vi "Main.vi"() -> ()   [LabVIEW 2012]
doc: "DESCRIPTION:\nThe One-Axis Move (Accel - Max Velocity - Decel) VI completes a move to user-specified position on a single axis while using user-specified acceleration, maximum velocity, and deceleration values. It also provides a monitor to track the progress of the move.\n\n*Note: This VI can be used as a subVI in a higher level program.\n\nINSTRUCTIONS:\n(1) Be sure your board is initialized before running this VI. Refer to the Initialization topic in the FlexMotion VI Online Help, which can be launched by choosing FlexMotion VI Online Help in the Help menu.\n\n(2) Select the Board ID that corresponds to your FlexMotion controller in the Board Configuration Utility. \n\n(3) Select the axis number to be used.\n\n(4) Set the Target Position (in encoder counts) to which you want the axis to move.\n\n(5) Set the values you wish to use for maximum velocity (RPM), acceleration (RPS/S), and deceleration (RPS/S).\n\n(6) Run the VI.\n\nKEY PARAMETERS:\n(1) Target Position: The position to which you want to move. This value needs to be changed every time you run the VI. If you run the VI twice in a row with the same target position, the motor will not move the second time since it will already be at its target position.\n\n(2) Velocity: The maximum velocity for the specified axis during the move.\n\n(3) Acceleration: The acceleration for the axis during the move.\n\n(4) Deceleration: The deceleration for the axis during the move. (This may be different than the acceleration.)\n\nI/O CONNECTIONS OVERVIEW:\nThis example requires a system configuration with one axis."
uses:
  MicroDrive.dll
panel:
  in  "Threshold(um)":dbl=0.5 format="%.3f"
  in  "Iterations":i32=1
  out "M6 Forward Limit":bool
  out "M6 Reverse Limit":bool
  out "M5 Forward Limit":bool
  out "M5 Reverse Limit":bool
  out "M4 Forward Limit":bool
  out "M4 Reverse Limit":bool
  in  "Reset M4":bool
  in  "Flip M4 Encoder":bool
  out "M4 Encoder (um)":dbl format="%.3f"
  in  "Flip M3 Encoder":bool
  in  "Flip M2 Encoder":bool
  in  "Flip M1 Encoder":bool
  out "M3 Encoder (um)":dbl format="%.3f"
  in  "Reset M3":bool
  out "M3 Forward Limit":bool
  out "M3 Reverse Limit":bool
  in  "Axis":enum16{"M1", "M2", "M3", "M4", "M5", "M6"}(ring)
  in  "Velocity (mm/s)":dbl=1.0 format="%.3f"
  in  "Move size (um)":dbl=50.0 format="%.3f"
  out "M2 Forward Limit":bool
  out "M2 Reverse Limit":bool
  out "M1 Forward Limit":bool
  out "M1 Reverse Limit":bool
  in  "stop":bool
  out "M2 Encoder (um)":dbl format="%.3f"
  in  "Reset  All":bool
  in  "Reset M2":bool
  out "M1 Encoder (um)":dbl format="%.3f"
  in  "Reset M1":bool
  in  "Move":bool
  in  "Stop":bool
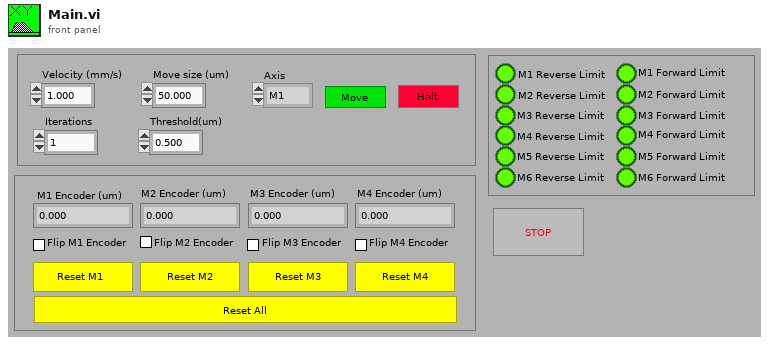
[diagram p1: front panel]
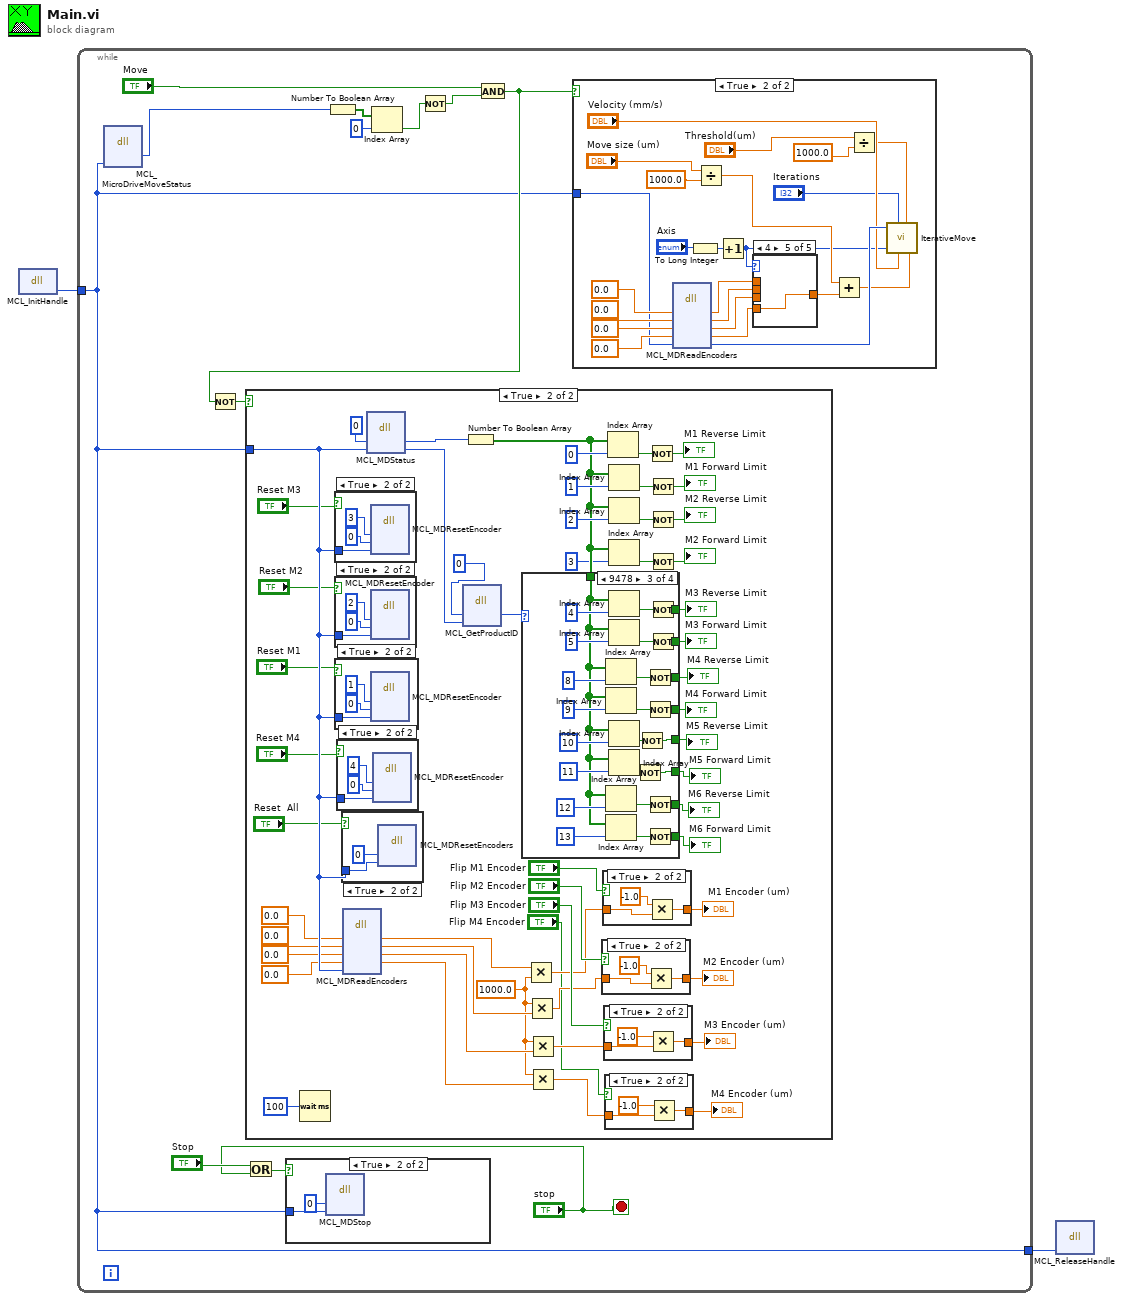
[diagram p0: block diagram]
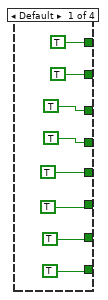
[diagram p9: hidden frame]
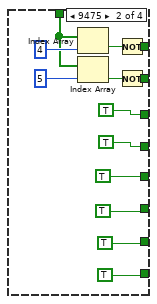
[diagram p10: hidden frame]
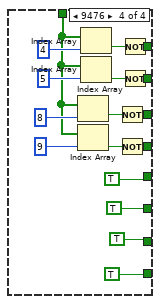
[diagram p11: hidden frame]
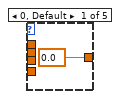
[diagram p17: hidden frame]
diagram:
  n1 = dll-call lib="C:/Users/Labview/Desktop/SRR/MicroDrive_x64/MicroDrive.dll" fn="MCL_InitHandle"() -> ("return type"=w2:i32)  [unwired: 3 in, 2 out]
  n2 = while {
    tunnel: w2 -> [w3]
    tunnel: [w3] -> w1
    stop <- "stop" stop-if-true
    n3 = dll-call lib="C:/Users/Labview/Desktop/SRR/MicroDrive_x64/MicroDrive.dll" fn="MCL_MicroDriveMoveStatus"("handle"=w3) -> ("isMoving"=w8:i32)  [unwired: 4 in, 4 out]
    n4 = Or(x="Stop", y="stop") -> (x .or. y?=w11:bool)
    n5 = case shown="True" w11 {
      tunnel: w3 -> [_ w15]
      frame False {
      }
      frame True {
        n6 = dll-call lib="C:/Users/Labview/Desktop/SRR/MicroDrive_x64/MicroDrive.dll" fn="MCL_MDStop"("status"=u16 0, "handle"=w15) -> ()  [unwired: 4 in, 4 out]
      }
    }
    n7 = Number To Boolean Array(number=w8) -> (Boolean array=w6:bool[])
    n8 = Index Array(array=w6, index=0) -> (element=w7:bool)
    n9 = Not(x=w7) -> (.not. x?=w9:bool)
    n10 = And(x="Move", y=w9) -> (x .and. y?=w4:bool)
    n11 = Not(x=w4) -> (.not. x?=w10:bool)
    n12 = case shown="True" w10 {
      tunnel: w3 -> [_ w57]
      frame False {
      }
      frame True {
        w36 = 1000.0
        n13 = Wait (ms)(milliseconds to wait=100) -> ()  [unwired: 1 out]
        n14 = case shown="True" "Reset M3" {
          tunnel: w57 -> [_ w72]
          frame False {
          }
          frame True {
            n15 = dll-call lib="C:/Users/Labview/Desktop/SRR/MicroDrive_x64/MicroDrive.dll" fn="MCL_MDResetEncoder"("axis"=u32 3, "status"=u16 0, "handle"=w72) -> ()  [unwired: 4 in, 5 out]
          }
        }
        n16 = case shown="True" "Reset M2" {
          tunnel: w57 -> [_ w75]
          frame False {
          }
          frame True {
            n17 = dll-call lib="C:/Users/Labview/Desktop/SRR/MicroDrive_x64/MicroDrive.dll" fn="MCL_MDResetEncoder"("axis"=u32 2, "status"=u16 0, "handle"=w75) -> ()  [unwired: 4 in, 5 out]
          }
        }
        n18 = case shown="True" "Reset M1" {
          tunnel: w57 -> [_ w78]
          frame False {
          }
          frame True {
            n19 = dll-call lib="C:/Users/Labview/Desktop/SRR/MicroDrive_x64/MicroDrive.dll" fn="MCL_MDResetEncoder"("axis"=u32 1, "status"=u16 0, "handle"=w78) -> ()  [unwired: 4 in, 5 out]
          }
        }
        n20 = case shown="True" "Reset M4" {
          tunnel: w57 -> [_ w81]
          frame False {
          }
          frame True {
            n21 = dll-call lib="C:/Users/Labview/Desktop/SRR/MicroDrive_x64/MicroDrive.dll" fn="MCL_MDResetEncoder"("axis"=u32 4, "status"=u16 0, "handle"=w81) -> ()  [unwired: 4 in, 5 out]
          }
        }
        n22 = case shown="True" "Reset  All" {
          tunnel: w57 -> [_ w83]
          frame False {
          }
          frame True {
            n23 = dll-call lib="C:/Users/Labview/Desktop/SRR/MicroDrive_x64/MicroDrive.dll" fn="MCL_MDResetEncoders"("status"=u16 0, "handle"=w83) -> ()  [unwired: 4 in, 4 out]
          }
        }
        n24 = dll-call lib="C:/Users/Labview/Desktop/SRR/MicroDrive_x64/MicroDrive.dll" fn="MCL_MDReadEncoders"("m1"=0.0, "m2"=0.0, "m3"=0.0, "m4"=0.0, "handle"=w57) -> ("m1"=w55:dbl, "m2"=w54:dbl, "m3"=w53:dbl, "m4"=w56:dbl)  [unwired: 4 in, 3 out]
        n25 = dll-call lib="C:/Users/Labview/Desktop/SRR/MicroDrive_x64/MicroDrive.dll" fn="MCL_MDStatus"("status"=u16 0, "handle"=w57) -> ("status"=w52:u16)  [unwired: 4 in, 3 out]
        n26 = dll-call lib="C:/Users/Labview/Desktop/SRR/MicroDrive_x64/MicroDrive.dll" fn="MCL_GetProductID"("PID"=u16 0, "handle"=w57) -> ("PID"=w37:u16)  [unwired: 4 in, 3 out]
        n27 = Number To Boolean Array(number=w52) -> (Boolean array=w58:bool[])
        n28 = case shown="9478" w37 {
          tunnel: [TRUE w103 w128 w145] -> w48
          tunnel: w58 -> [_ w101 w105 w134]
          tunnel: [TRUE w99 w125 w142] -> w47
          tunnel: [TRUE TRUE w111 w136] -> w32
          tunnel: [TRUE TRUE w110 w135] -> w31
          tunnel: [TRUE TRUE w109 TRUE] -> w30
          tunnel: [TRUE TRUE w108 TRUE] -> w29
          tunnel: [TRUE TRUE w107 TRUE] -> w28
          tunnel: [TRUE TRUE w106 TRUE] -> w27
          frame Default {
          }
          frame 9475 {
            n29 = Index Array(array=w101, index=4) -> (element=w104:bool)
            n30 = Index Array(array=w101, index=5) -> (element=w98:bool)
            n31 = Not(x=w104) -> (.not. x?=w103:bool)
            n32 = Not(x=w98) -> (.not. x?=w99:bool)
          }
          frame 9478 {
            n33 = Index Array(array=w105, index=8) -> (element=w123:bool)
            n34 = Index Array(array=w105, index=9) -> (element=w120:bool)
            n35 = Index Array(array=w105, index=12) -> (element=w115:bool)
            n36 = Index Array(array=w105, index=13) -> (element=w112:bool)
            n37 = Index Array(array=w105, index=4) -> (element=w129:bool)
            n38 = Index Array(array=w105, index=5) -> (element=w124:bool)
            n39 = Index Array(array=w105, index=10) -> (element=w119:bool)
            n40 = Index Array(array=w105, index=11) -> (element=w116:bool)
            n41 = Not(x=w116) -> (.not. x?=w108:bool)
            n42 = Not(x=w119) -> (.not. x?=w109:bool)
            n43 = Not(x=w123) -> (.not. x?=w111:bool)
            n44 = Not(x=w120) -> (.not. x?=w110:bool)
            n45 = Not(x=w115) -> (.not. x?=w107:bool)
            n46 = Not(x=w112) -> (.not. x?=w106:bool)
            n47 = Not(x=w129) -> (.not. x?=w128:bool)
            n48 = Not(x=w124) -> (.not. x?=w125:bool)
          }
          frame 9476 {
            n49 = Index Array(array=w134, index=8) -> (element=w140:bool)
            n50 = Index Array(array=w134, index=9) -> (element=w137:bool)
            n51 = Index Array(array=w134, index=4) -> (element=w146:bool)
            n52 = Index Array(array=w134, index=5) -> (element=w141:bool)
            n53 = Not(x=w140) -> (.not. x?=w136:bool)
            n54 = Not(x=w137) -> (.not. x?=w135:bool)
            n55 = Not(x=w146) -> (.not. x?=w145:bool)
            n56 = Not(x=w141) -> (.not. x?=w142:bool)
          }
        }
        "M3 Reverse Limit" <- w48
        "M3 Forward Limit" <- w47
        "M4 Forward Limit" <- w31
        "M5 Reverse Limit" <- w30
        "M5 Forward Limit" <- w29
        "M6 Reverse Limit" <- w28
        "M6 Forward Limit" <- w27
        "M4 Reverse Limit" <- w32
        n57 = Multiply(x=w55, y=w36) -> (x*y=w39:dbl)
        n58 = Multiply(x=w36, y=w54) -> (x*y=w42:dbl)
        n59 = Multiply(x=w36, y=w53) -> (x*y=w46:dbl)
        n60 = Multiply(x=w36, y=w56) -> (x*y=w35:dbl)
        n61 = case shown="True" "Flip M2 Encoder" {
          tunnel: w42 -> [w151 w153]
          tunnel: [w151 w154] -> w43
          frame False {
          }
          frame True {
            n62 = Multiply(x=-1.0, y=w153) -> (x*y=w154:dbl)
          }
        }
        "M2 Encoder (um)" <- w43
        n63 = case shown="True" "Flip M1 Encoder" {
          tunnel: w39 -> [w147 w149]
          tunnel: [w147 w150] -> w40
          frame False {
          }
          frame True {
            n64 = Multiply(x=-1.0, y=w149) -> (x*y=w150:dbl)
          }
        }
        "M1 Encoder (um)" <- w40
        n65 = case shown="True" "Flip M3 Encoder" {
          tunnel: w46 -> [w155 w157]
          tunnel: [w155 w158] -> w44
          frame False {
          }
          frame True {
            n66 = Multiply(x=-1.0, y=w157) -> (x*y=w158:dbl)
          }
        }
        "M3 Encoder (um)" <- w44
        n67 = case shown="True" "Flip M4 Encoder" {
          tunnel: w35 -> [w159 w161]
          tunnel: [w159 w162] -> w34
          frame False {
          }
          frame True {
            n68 = Multiply(x=-1.0, y=w161) -> (x*y=w162:dbl)
          }
        }
        "M4 Encoder (um)" <- w34
        n69 = Index Array(array=w58, index=0) -> (element=w62:bool)
        n70 = Index Array(array=w58, index=1) -> (element=w63:bool)
        n71 = Index Array(array=w58, index=2) -> (element=w64:bool)
        n72 = Index Array(array=w58, index=3) -> (element=w50:bool)
        n73 = Not(x=w62) -> (.not. x?=→"M1 Reverse Limit":bool)
        n74 = Not(x=w63) -> (.not. x?=→"M1 Forward Limit":bool)
        n75 = Not(x=w64) -> (.not. x?=→"M2 Reverse Limit":bool)
        n76 = Not(x=w50) -> (.not. x?=→"M2 Forward Limit":bool)
      }
    }
    n77 = case shown="True" w4 {
      tunnel: w3 -> [_ w177]
      frame False {
      }
      frame True {
        n78 = dll-call lib="C:/Users/Labview/Desktop/SRR/MicroDrive_x64/MicroDrive.dll" fn="MCL_MDReadEncoders"("m1"=0.0, "m2"=0.0, "m3"=0.0, "m4"=0.0, "handle"=w177) -> ("m1"=w175:dbl, "m2"=w174:dbl, "m3"=w173:dbl, "m4"=w172:dbl, "handle"=w176:i32)  [unwired: 3 in, 3 out]
        n79 = To Long Integer(number="Axis") -> (32bit integer=w182:i32)
        n80 = Divide(x="Move size (um)", y=1000.0) -> (x/y=w170:dbl)
        n81 = Increment(x=w182) -> (x+1=w167:i32)
        n82 = case shown="4" w167 {
          tunnel: w175 -> [_ w187 _ _ _]
          tunnel: w174 -> [_ _ w188 _ _]
          tunnel: w173 -> [_ _ _ w189 _]
          tunnel: w172 -> [_ _ _ _ w190]
          tunnel: [0.0 w187 w188 w189 w190] -> w171
          frame 0, Default {
          }
          frame 1 {
          }
          frame 2 {
          }
          frame 3 {
          }
          frame 4 {
          }
        }
        n83 = Add(x=w170, y=w171) -> (x+y=w169:dbl)
        n84 = Divide(x="Threshold(um)", y=1000.0) -> (x/y=w164:dbl)
        n85 = call "IterativeMove.vi"("Handle"=w176, "IterativeMoves"="Iterations", "Axis"=w167, "Velocity"="Velocity (mm/s)", "Threshold (mm)"=w164, "Goal"=w169) -> ()  [unwired: 4 in]
      }
    }
  }
  n86 = dll-call lib="C:/Users/Labview/Desktop/SRR/MicroDrive_x64/MicroDrive.dll" fn="MCL_ReleaseHandle"("handle"=w1) -> ()  [unwired: 4 in, 3 out]
